vi "From JSON Tree.vi"(8 "error in (no error)":errorcluster, 10 "JSON Tree In":variant, 11 "id in":refnum<class "id.lvclass">) -> (0 "error out":errorcluster, 3 "id out":refnum<class "id.lvclass">)   [LabVIEW 2015, in "id.lvclass"]
uses:
  id.lvclass
  <vilib>/rajsite/i3-json/JSON Types/JSON Type.ctl
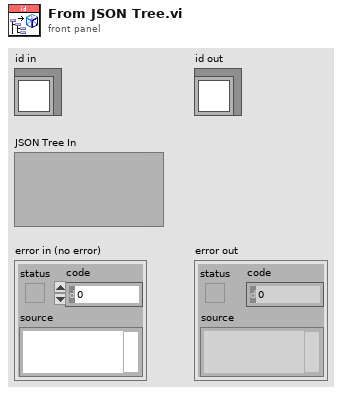
[diagram p1: front panel]
types:
  T1 = typedef "i3-json.lvlib/JSON Type.ctl" = enum8{"JSON Compatible", "JSON Array", "JSON Object", "JSON Null", "Double", "String", "Boolean", "Unknown"}
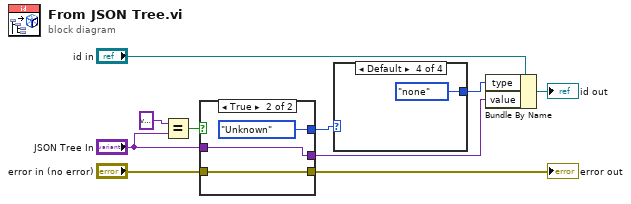
[diagram p0: block diagram]
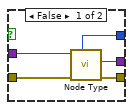
[diagram p2: hidden frame]
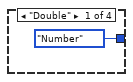
[diagram p3: hidden frame]
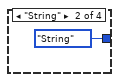
[diagram p4: hidden frame]
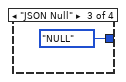
[diagram p5: hidden frame]
diagram:
  n1 = Equal?(x=variant, y="JSON Tree In") -> (x = y?=w1:bool)
  n2 = case shown="True" w1 {
    tunnel: [w15 w17] -> w8
    tunnel: [w14 JSON_Type."Unknown" ("JSON Type")] -> w7
    tunnel: "error in (no error)" -> [w13 w16]
    tunnel: [w12 w16] -> w4
    tunnel: "JSON Tree In" -> [w11 w17]
    frame False {
      n3 = call <vilib>:"Node Type.vi"("error in (no error)"=w13, "JSON Tree In"=w11) -> ("error out"=w12:errorcluster, "Value"=w15:variant, "JSON Type"=w14:T1)  [unwired: 5 in, 2 out]
    }
    frame True {
    }
  }
  "error out" <- w4
  n4 = case shown="Default" w7 {
    tunnel: [enum16{"none", "String", "Number", "NULL"}."Number" ("type") enum16{"none", "String", "Number", "NULL"}."String" ("type") enum16{"none", "String", "Number", "NULL"}."NULL" ("type") enum16{"none", "String", "Number", "NULL"}."none" ("type")] -> w6
    frame "Double" {
    }
    frame "String" {
    }
    frame "JSON Null" {
    }
    frame Default {
    }
  }
  n5 = Bundle By Name(cluster="id in", "type"=w6, "value"=w8) -> (→"id out":refnum<class "id.lvclass">)
